vi "Close.vi"(8 "ErrorIn":errorcluster, 11 "VISAIn":refnum<visa-resource-name>) -> (0 "ErrorOut":errorcluster)   [LabVIEW 2017, in "I28Drivers.lvlib"]
uses:
  I28Drivers.lvlib
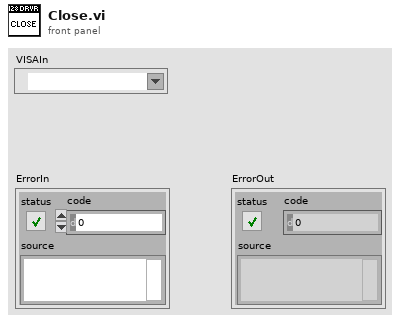
[diagram p1: front panel]
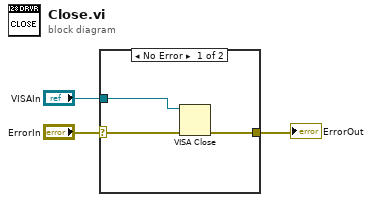
[diagram p0: block diagram]
diagram:
  n1 = case shown="No Error" "ErrorIn" {
    selector: "ErrorIn" -> [w5 w7]
    tunnel: "VISAIn" -> [w6 _]
    tunnel: [w4 w7] -> w1
    frame No Error {
      n2 = VISA Close(VISA resource name=w6, error in (no error)=w5) -> (error out=w4:errorcluster)
    }
    frame Error {
    }
  }
  "ErrorOut" <- w1
